vi "Initialization VI.vi"(8 "error in (no error)":errorcluster, 10 "Custom XML":string, 11 "Device Item Ref in":T1 format="%.0x") -> (0 "error out":errorcluster, 3 "Device Item Ref out":T1 format="%.0x")   [LabVIEW 2023, in "Waveform Analog Output System Explorer.lvlib"]
uses:
  Waveform Analog Output System Explorer.lvlib
  <vilib>/NI VeriStand/Custom Device API/Custom Device Item Ref.ctl
  <vilib>/NI VeriStand/Custom Device API/Custom Device Channel.ctl
  <vilib>/NI VeriStand/Custom Device API/Custom Device Channel Type.ctl
  Shared/Constants.vi
  <vilib>/NI VeriStand/Custom Device API/Set Item Property (Variant).vi
  <vilib>/NI VeriStand/Custom Device API/Custom Device API.lvlib
  Shared/Waveform Analog Output Shared.lvlib
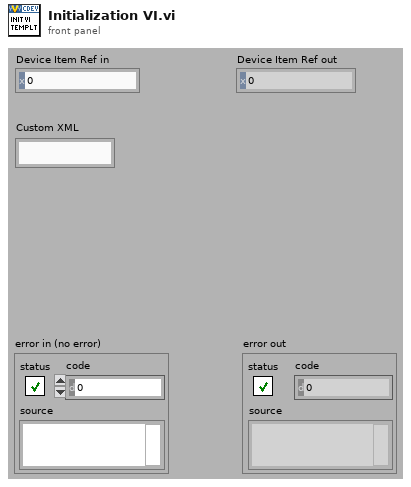
[diagram p1: front panel]
types:
  T1 = typedef "Custom Device API.lvlib/Custom Device Item Ref.ctl" = u64
  T2 = typedef "Custom Device API.lvlib/Custom Device Channel.ctl" = cluster{"Type":T3, "Units":string, "Default Value":dbl, "Faultable":bool, "Scalable":bool}
  T3 = typedef "Custom Device API.lvlib/Custom Device Channel Type.ctl" = enum16{"Input", "Output"}
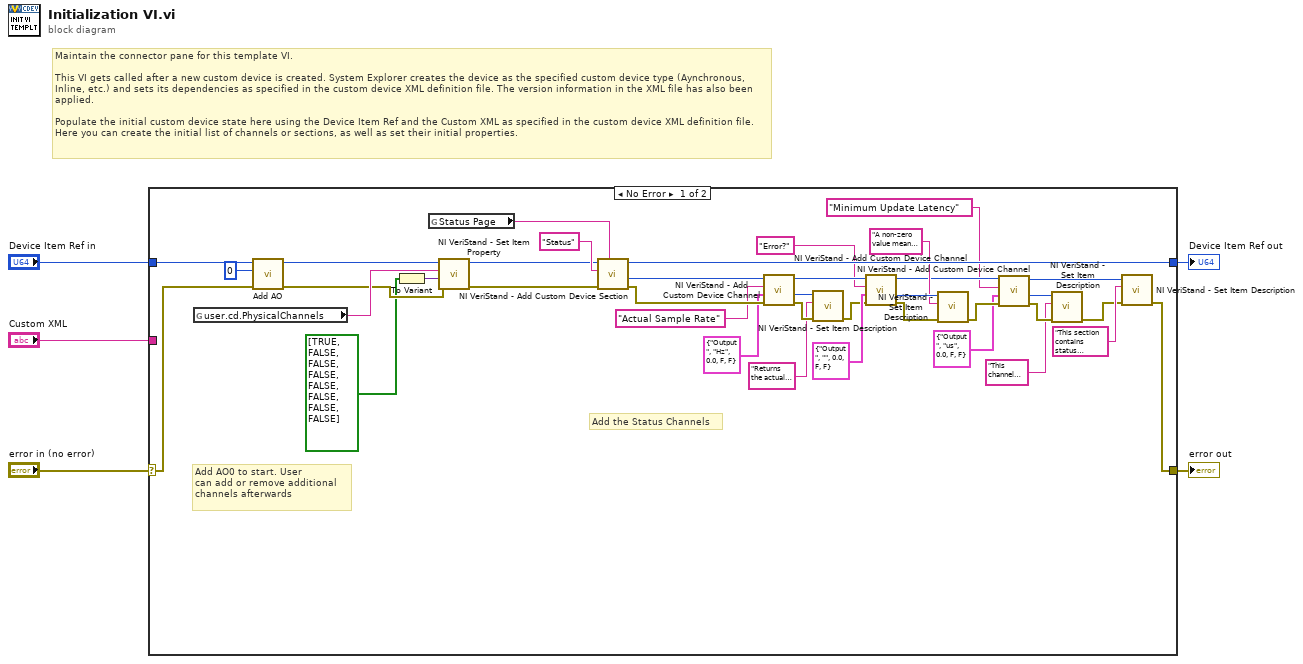
[diagram p0: block diagram]
diagram:
  # "Maintain the connector pane for this template VI.\n\nThis VI gets called after a new custom device is created. System Explorer creates the device as the specified custom device type (Aynchronous, Inline, etc.) and sets its dependencies as specified in the custom device XML definition file. The version information in the XML file has also been applied.\n\nPopulate the initial custom device state here using the Device Item Ref and the Custom XML as specified in the custom device XML definition file. Here you can create the initial list of channels or sections, as well as set their initial properties."
  n1 = case shown="No Error" "error in (no error)" {
    selector: "error in (no error)" -> [w42 w45]
    tunnel: [w16 w45] -> w5
    tunnel: [w39 w44] -> w3
    tunnel: "Device Item Ref in" -> [w43 w44]
    tunnel: "Custom XML" -> [_ _]
    frame No Error {
      # "Add the Status Channels"
      # "Add AO0 to start. User\ncan add or remove additional\nchannels afterwards"
      n2 = global read "Constants.vi" "user.cd.PhysicalChannels"() -> (w34:string)
      n3 = call "Add AO.vi"("error in (no error)"=w42, "Physical Channel Number"=0, "Device Item Ref in"=w43) -> ("error out"=w30:errorcluster, "Parent Ref out"=w32:T1)  [unwired: 7 in]
      n4 = To Variant(anything=bool[] [TRUE, FALSE, FALSE, FALSE, FALSE, FALSE, FALSE, FALSE]) -> (Variant=w33:variant)
      n5 = global read "Constants.vi" "Status Page"() -> (w15:string)
      n6 = call-poly <vilib>:"NI VeriStand - Set Item Property.vi"("error in (no error)"=w30, "Value"=w33, "Property Name"=w34, "Item Ref in"=w32) -> ("error out"=w29:errorcluster, "Item Ref out"=w31:T1)  [unwired: 5 in, 1 out]
      n7 = call <vilib>:"NI VeriStand - Add Custom Device Section.vi"("GUID (Default Section)"=w15, "error in (no error)"=w29, "Section Name"="Status", "Parent Ref in"=w31) -> ("error out"=w37:errorcluster, "Section Ptr"=w38:T1, "Parent Ref out"=w39:T1)  [unwired: 4 in, 1 out]
      n8 = call <vilib>:"NI VeriStand - Add Custom Device Channel.vi"("error in (no error)"=w37, "Channel"=T2 {"Type"=enum."Output", "Units"="Hz", "Default Value"=0.0, "Faultable"=FALSE, "Scalable"=FALSE}, "Channel Name"="Actual Sample Rate", "Parent Ref in"=w38) -> ("error out"=w20:errorcluster, "Channel Ref"=w21:T1, "Parent Ref out"=w27:T1)  [unwired: 4 in, 1 out]
      n9 = call <vilib>:"NI VeriStand - Set Item Description.vi"("error in (no error)"=w20, "Description"="Returns the actual sample rate that the DAQ card is using to generate the waveforms. This value is returned during initialization and will not change as the system runs.", "Item Ref in"=w21) -> ("error out"=w19:errorcluster)  [unwired: 6 in, 2 out]
      n10 = call <vilib>:"NI VeriStand - Add Custom Device Channel.vi"("error in (no error)"=w19, "Channel"=T2 {"Type"=enum."Output", "Units"="", "Default Value"=0.0, "Faultable"=FALSE, "Scalable"=FALSE}, "Channel Name"="Error?", "Parent Ref in"=w27) -> ("error out"=w23:errorcluster, "Channel Ref"=w24:T1, "Parent Ref out"=w14:T1)  [unwired: 4 in, 1 out]
      n11 = call <vilib>:"NI VeriStand - Set Item Description.vi"("error in (no error)"=w23, "Description"="A non-zero value means an error has occurred and the custom device has shut down", "Item Ref in"=w24) -> ("error out"=w13:errorcluster)  [unwired: 6 in, 2 out]
      n12 = call <vilib>:"NI VeriStand - Add Custom Device Channel.vi"("error in (no error)"=w13, "Channel"=T2 {"Type"=enum."Output", "Units"="us", "Default Value"=0.0, "Faultable"=FALSE, "Scalable"=FALSE}, "Channel Name"="Minimum Update Latency", "Parent Ref in"=w14) -> ("error out"=w9:errorcluster, "Channel Ref"=w10:T1, "Parent Ref out"=w7:T1)  [unwired: 4 in, 1 out]
      n13 = call <vilib>:"NI VeriStand - Set Item Description.vi"("error in (no error)"=w9, "Description"="This channel outputs the minimum latency expected for new parameter values to update the waveform. This latency is calculated based on the current write location in the output buffer when a parameter value change occurs. Note that the latency can be slightly higher based on write location of the HW buffer.", "Item Ref in"=w10) -> ("error out"=w6:errorcluster)  [unwired: 6 in, 2 out]
      n14 = call <vilib>:"NI VeriStand - Set Item Description.vi"("error in (no error)"=w6, "Description"="This section contains status channels useful for tracking the health of this custom device.", "Item Ref in"=w7) -> ("error out"=w16:errorcluster)  [unwired: 6 in, 2 out]
    }
    frame Error {
    }
  }
  "error out" <- w5
  "Device Item Ref out" <- w3
